vi "Execute.vi"(8 "error in (no error)":errorcluster, 10 "ObserverRegistry in":refnum<class "ObserverRegistry.lvclass">, 11 "ObserverRegistryCommand":refnum<class "Observer_RegisterByLabel.lvclass">) -> (0 "error out":errorcluster, 2 "ObserverRegistry out":refnum<class "ObserverRegistry.lvclass">, 3 "Message":refnum<class "MSG.lvclass">)   [LabVIEW 2011, in "Messenging.lvlib" / "Observer_RegisterByLabel.lvclass"]
uses:
  Observer_RegisterByLabel.lvclass
  ObserverRegistry.lvclass
  Messenging.lvlib
  Interprocess Messenger/SendMultiple/Create Observer.vi
  Interprocess Messenger/SendMultiple/ObserverSet.lvclass
  ParentCommand/ObserverRegistryCommand.lvclass
  Interprocess Messenger/TextVarientMessage/MSG.lvclass
  Registration Entry.ctl
  Interprocess Messenger/SendOnly/Observer.lvclass
  Interprocess Messenger/Send/Send.lvclass
  Interprocess Messenger/Send/Send Message.vi
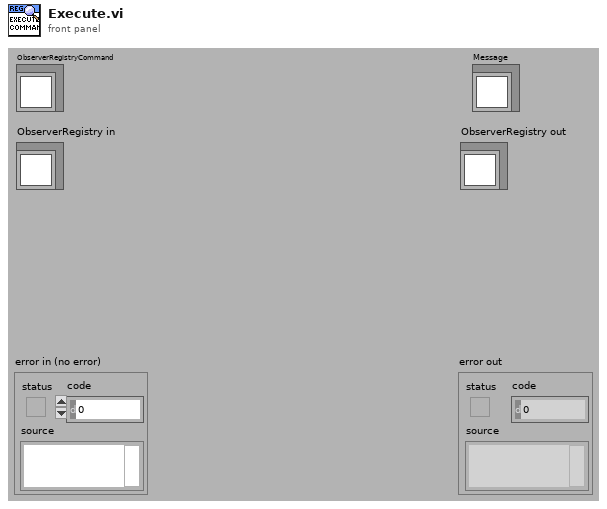
[diagram p1: front panel]
types:
  T1 = typedef "Messenging.lvlib/ObserverRegistry.lvclass/Registration Entry.ctl" = cluster{"Observer":refnum<class "Observer.lvclass">, "Type":enum16{"Event", "State"}, "Latest (State)":refnum<class "MSG.lvclass">}
  T2 = typedef "Messenging.lvlib/ObserverRegistry.lvclass/ObserverRegistryData.ctl" = cluster{"Observer of Errors":refnum<class "Observer.lvclass">, "Observer of All":refnum<class "Observer.lvclass">, "Event Registry":variant}
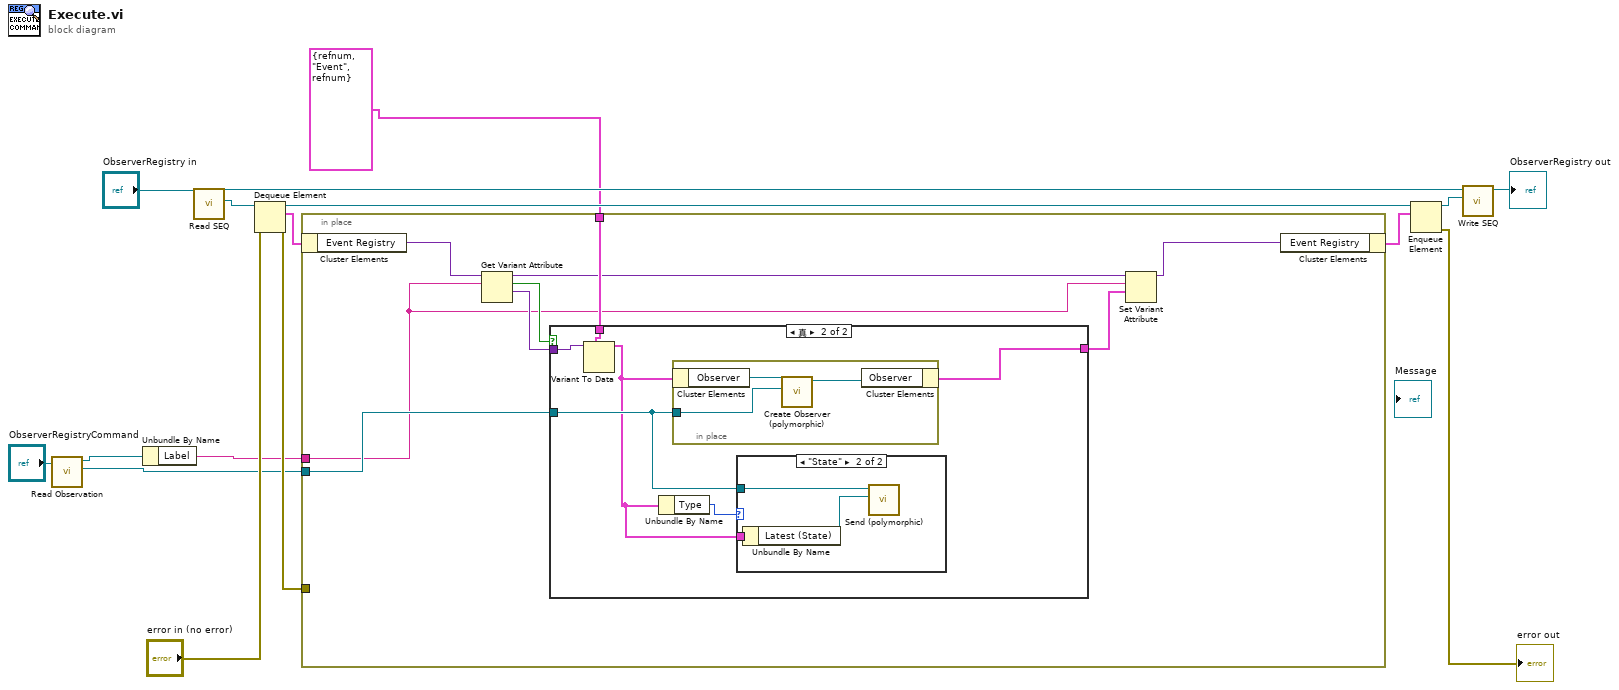
[diagram p0: block diagram]
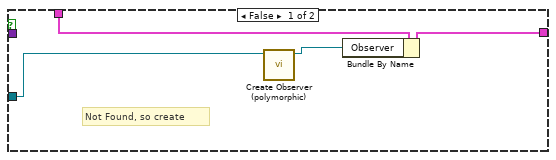
[diagram p2: hidden frame]
diagram:
  n1 = call "Read Observation.vi"("ObserverRegistryCommand.lvclass in"="ObserverRegistryCommand") -> ("Observer"=w3:refnum<class "Send.lvclass">, "ObserverRegistryCommand.lvclass out"=w2:refnum<class "Observer_RegisterByLabel.lvclass">)  [unwired: 1 in, 8 out]
  n2 = Unbundle By Name(w2) -> ("Label"=w1:string)
  n3 = call "Read SEQ.vi"("ObserverRegistry.lvclass in"="ObserverRegistry in") -> ("SEQ"=w9:refnum<queue>, "ObserverRegistry.lvclass out"=w7:refnum<class "ObserverRegistry.lvclass">)  [unwired: 1 in, 8 out]
  n4 = Dequeue Element(queue=w9, error in (no error)="error in (no error)") -> (queue out=w14:refnum<queue>, element=w16:T2, error out=w12:errorcluster)  [unwired: 2 out]
  n5 = in-place {
    in-place-border: w12 -> [_]
    in-place-border: w1 -> [w18]
    in-place-border: w3 -> [w21]
    in-place-border: T1 {"Observer"=refnum, "Type"=enum."Event", "Latest (State)"=refnum} ("Registration Entry") -> [w22]
    n6 = in-place-cluster #1(w16) -> ("Event Registry"=w25:variant)
    n7 = Get Variant Attribute(Variant=w25, name=w18) -> (duplicate Variant=w19:variant, found=w24:bool, value=w23:variant)  [unwired: 2 in, 1 out]
    n8 = case shown="真" w24 {
      tunnel: w23 -> [_ w35]
      tunnel: w22 -> [w29 w34]
      tunnel: w21 -> [w26 w31]
      tunnel: [w28 w33] -> w20
      frame False {
        # "Not Found, so create"
        n9 = call-poly "Create Observer (polymorphic).vi"("Input"=w26) -> ("Observer"=w27:refnum<class "Observer.lvclass">)  [unwired: 8 out]
        n10 = Bundle By Name(cluster=w29, "Observer"=w27) -> (w28:T1)
      }
      frame True {
        n11 = Variant To Data(type=w34, Variant=w35) -> (data=w30:T1)  [unwired: 1 in, 1 out]
        n12 = Unbundle By Name(w30) -> ("Type"=w32:enum16{"Event", "State"})
        n13 = in-place {
          in-place-border: w31 -> [w39]
          n14 = in-place-cluster #2(w30) -> ("Observer"=w41:refnum<class "Observer.lvclass">)
          n15 = call-poly "Create Observer (polymorphic).vi"("Additional Input"=w39, "Input"=w41) -> ("Observer"=w40:refnum<class "Observer.lvclass">)  [unwired: 7 out]
          n16 = in-place-cluster #2("Observer"=w40) -> (w33:T1)
        }
        n17 = case shown="\"State\"" w32 {
          tunnel: w31 -> [_ w38]
          tunnel: w30 -> [_ w37]
          frame "Event", Default {
          }
          frame "State" {
            n18 = Unbundle By Name(w37) -> ("Latest (State)"=w36:refnum<class "MSG.lvclass">)
            n19 = call-poly "Send (polymorphic).vi"("Message"=w36, "MSR Parent in"=w38) -> ()  [unwired: 1 in, 9 out]
          }
        }
      }
    }
    n20 = Set Variant Attribute(Variant=w19, name=w18, value=w20) -> (Variant out=w17:variant)  [unwired: 1 in, 2 out]
    n21 = in-place-cluster #1("Event Registry"=w17) -> (w15:T2)
  }
  n22 = Enqueue Element(queue=w14, element=w15) -> (queue out=w6:refnum<queue>, error out=→"error out":errorcluster)  [unwired: 1 in, 2 out]
  n23 = call "Write SEQ.vi"("SEQ"=w6, "ObserverRegistry.lvclass in"=w7) -> ("ObserverRegistry.lvclass out"=→"ObserverRegistry out":refnum<class "ObserverRegistry.lvclass">)  [unwired: 1 in, 8 out]
